vi "Analise Fell Rock.vi"(0 "Chamber":u32[][](array[colorbox])=array3069x7[21483 elements]) -> ()   [LabVIEW 2020, in "AoC 2022.lvlib"]
uses:
  AoC 2022.lvlib
panel:
  out "Chamber 3":u32[][](array[colorbox])
  out "Chamber 2":u32[][](array[colorbox])
  out "Chamber 1":u32[][](array[colorbox])
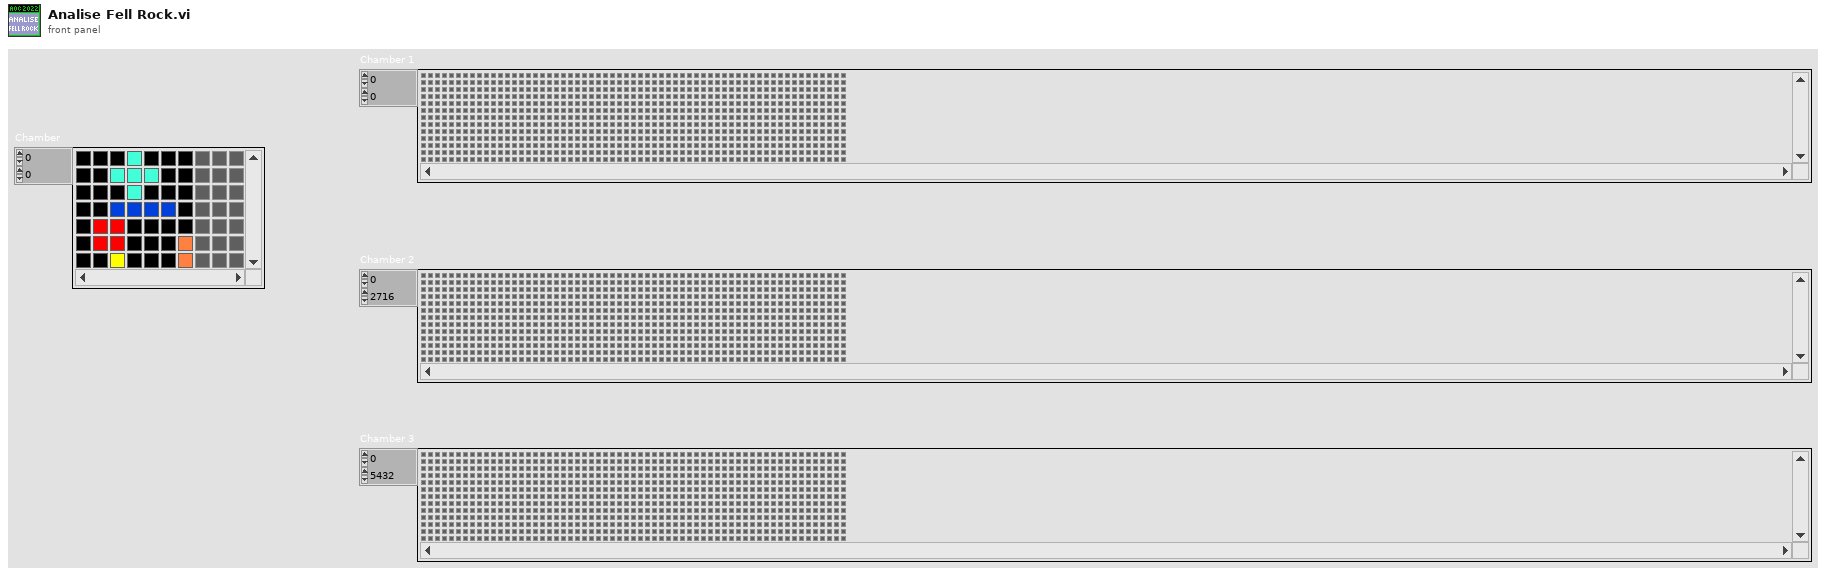
[diagram p1: front panel]
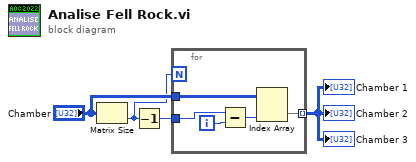
[diagram p0: block diagram]
diagram:
  n1 = Matrix Size(0:"Chamber") -> (2:w3:i32)  [unwired: 1 out]
  n2 = Decrement(x=w3) -> (x-1=w2:i32)
  n3 = for {
    N: w3 -> [_]
    tunnel: "Chamber" -> [w9]
    tunnel: [w7] -> w1 mode=indexing
    tunnel: w2 -> [w5]
    i -> [w8]
    n4 = Subtract(x=w5, y=w8) -> (x-y=w6:i32)
    n5 = Index Array(array=w9, index (col)=w6) -> (element=w7:u32[])  [unwired: 1 in]
  }
  "Chamber 1" <- w1
  "Chamber 2" <- w1
  "Chamber 3" <- w1
